vi "关闭连接.vi"(8 "error in":errorcluster, 11 "TCP Connection Ref":refnum<k5>) -> (0 "error out":errorcluster)   [LabVIEW 2017]
uses:
  S7 TCP API Library/S7 TCP.lvlib
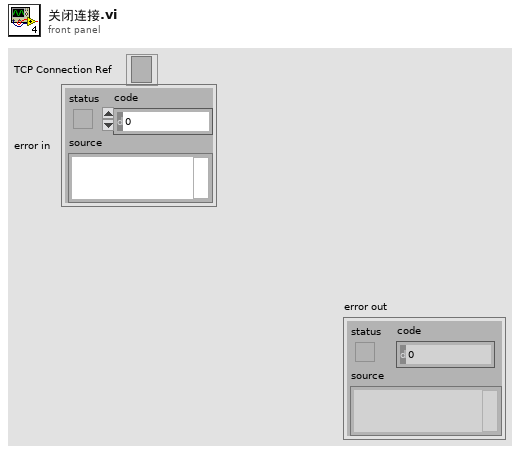
[diagram p1: front panel]
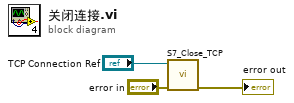
[diagram p0: block diagram]
diagram:
  n1 = call "S7_Close_TCP.vi"("error in"="error in", "TCP Connection Ref"="TCP Connection Ref") -> ("error out"=→"error out":errorcluster)  [unwired: 1 in, 8 out]
